vi "求面积.vi"(1 "Image":T1) -> (0 "数值输入控件":dbl)   [LabVIEW 2018]
uses:
  <vilib>/vision/Image Controls.llb/IMAQ Image.ctl
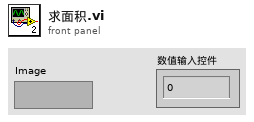
[diagram p1: front panel]
types:
  T1 = typedef "IMAQ Image.ctl" = refnum<image>
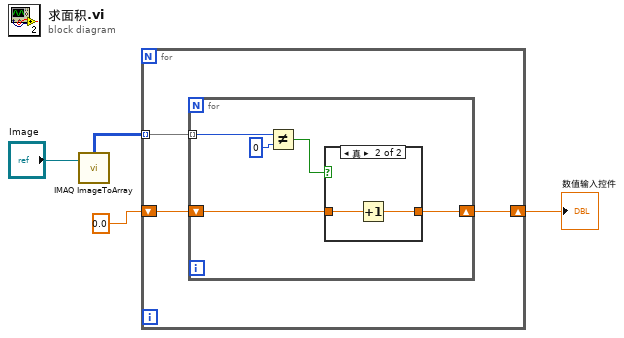
[diagram p0: block diagram]
diagram:
  n1 = call "IMAQ ImageToArray"("Image"="Image") -> ("Image Pixels (U8)"=w3:u8[][])  [unwired: 3 in, 4 out]
  n2 = for {
    tunnel: w3 -> [w7] mode=indexing
    shift-right: [w5] -> w1
    shift-left: 0.0 -> [w6]
    n3 = for {
      tunnel: w7 -> [w12] mode=indexing
      shift-right: [w9] -> w5
      shift-left: w6 -> [w10]
      n4 = Not Equal?(x=w12, y=u8 0) -> (x != y?=w8:bool)
      n5 = case shown="真" w8 {
        tunnel: w10 -> [w13 w15]
        tunnel: [w13 w14] -> w9
        frame False {
        }
        frame True {
          n6 = Increment(x=w15) -> (x+1=w14:dbl)
        }
      }
    }
  }
  "数值输入控件" <- w1
